vi "Rotate.vi"(7 "Transform Matrix":dbl[][](array[numeric])=[[1.0, 0.0], [0.0, 1.0]], 10 "Y":dbl, 11 "X":dbl) -> (0 "error out":errorcluster, 2 "Yrot":dbl, 3 "Xrot":dbl)   [LabVIEW 2014]
uses:
  <vilib>/Analysis/Matrix/Numeric/Conversions/Array To Matrix - RA2.vi
  <vilib>/Analysis/Matrix/Numeric/Multiply/Multiply - RM,RM.vi
  <vilib>/Analysis/Matrix/Numeric/Conversions/Matrix To Array - RM.vi
  <vilib>/Analysis/Matrix/NI_Matrix.lvlib
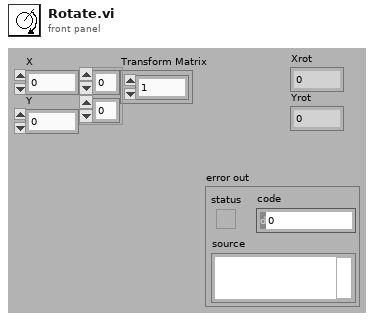
[diagram p1: front panel]
types:
  T1 = typedef "NI_Matrix.lvlib/RealMatrix.ctl" = dbl[][]
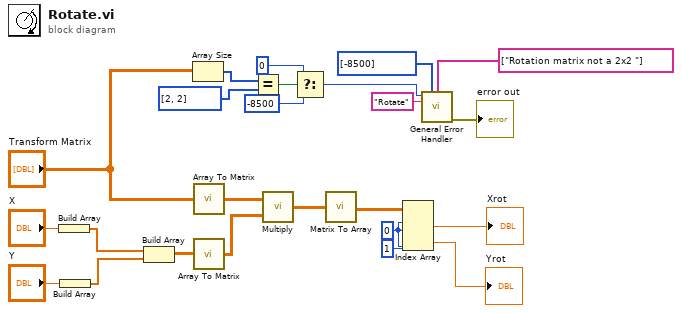
[diagram p0: block diagram]
diagram:
  w6 = 0 ("disabled index (col)")
  n1 = Build Array("X") -> (w10:dbl[])
  n2 = Build Array("Y") -> (w12:dbl[])
  n3 = Build Array(w10, w12) -> (w9:dbl[][])
  n4 = Array Size(array="Transform Matrix") -> (size(s)=w23:i32[])
  n5 = call-poly <vilib>:"Array To Matrix.vi"("Real 2D Array"="Transform Matrix") -> ("Real Matrix"=w1:T1)
  n6 = call-poly <vilib>:"Array To Matrix.vi"("Real 2D Array"=w9) -> ("Real Matrix"=w2:T1)
  n7 = Equal?(x=w23, y=i32[] [2, 2]) -> (x = y?=w17:bool)
  n8 = call-poly <vilib>:"Multiply.vi"("Real Matrix B"=w2, "Real Matrix A"=w1) -> ("A * B"=w8:T1)
  n9 = Select(t=0, s=w17, f=-8500) -> (s? t:f=w14:i32)
  n10 = call-poly <vilib>:"Matrix To Array.vi"("Real Matrix"=w8) -> ("Real 2D Array"=w7:dbl[][])
  n11 = Index Array(array=w7, index (row) #1=w6, index (col) #1=w6, index (row) #2=1 ("disabled index (row)"), index (col) #2=w6) -> (element #1=→"Xrot":dbl, element #2=→"Yrot":dbl)
  n12 = call <vilib>:"General Error Handler.vi"("[error code] (0)"=w14, "[user-defined codes]"=i32[] [-8500], "[user-defined descriptions]"=string[] ["Rotation matrix not a 2x2 "], "[error source] (\" \")"="Rotate" ("[error source] (\" \")")) -> ("error out"=→"error out":errorcluster)  [unwired: 7 in, 4 out]
